vi "XL320_Change Motor ID.vi"(8 "error in (no error)":errorcluster, 9 "New ID":u8, 10 "Current ID":u8, 11 "VISA resource name":refnum<visa-resource-name>) -> (0 "error out":errorcluster, 3 "VISA Resource Out":refnum<visa-resource-name>)   [LabVIEW 2017, in "Dynamixel XL320.lvlib"]
doc: "Changes a motor's ID."
uses:
  <instrlib>/Dynamixel XL320 (Drivers instrument)/Dynamixel XL320.lvlib
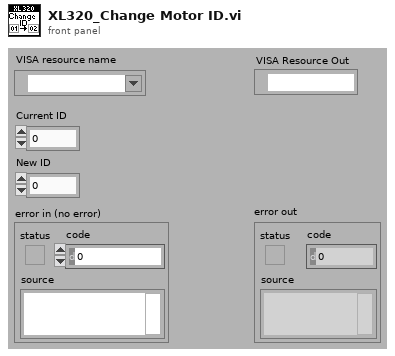
[diagram p1: front panel]
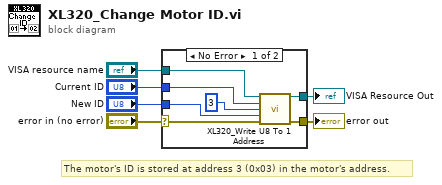
[diagram p0: block diagram]
diagram:
  # "The motor's ID is stored at address 3 (0x03) in the motor's address."
  n1 = case shown="No Error" "error in (no error)" {
    selector: "error in (no error)" -> [w9 w15]
    tunnel: [w8 w15] -> w3
    tunnel: [w7 w14] -> w2
    tunnel: "VISA resource name" -> [w13 w14]
    tunnel: "Current ID" -> [w12 _]
    tunnel: "New ID" -> [w10 _]
    frame No Error {
      n2 = call <instrlib>:"XL320_Write U8 To 1 Address.vi"("VISA resource name"=w13, "Motor ID (0)"=w12, "Address number (0)"=u16 3 ("Address"), "Parameter (0)"=w10, "error in (no error)"=w9) -> ("VISA resource name out"=w7:refnum<visa-resource-name>, "error out"=w8:errorcluster)  [unwired: 9 in]
    }
    frame Error {
    }
  }
  "error out" <- w3
  "VISA Resource Out" <- w2
